vi "ScientiFic DC Power Supply Output DC Volts.vi"() -> ()   [LabVIEW 2020]
doc: "This example shows how to configure the instrument's output voltage level, over current protection, and over voltage protection. The actual voltage level and actual current level are returned as well as whether over voltage protection (OVP) or over current protection (OCP) has been tripped."
uses:
  <instrlib>/ScientiFic DC Power Supply/Public/Ch Selector.ctl
  <instrlib>/ScientiFic DC Power Supply/ScientiFic DC Power Supply.lvlib
panel:
  in  "Ch Selector":T1
  in  "Serial Configuration":T2={"Baud Rate"=9600, "Parity"=0, "Data Bits"=8, "Stop Bits"=10, "Flow Control"=0, "Remote Channel"="CH 1"} {"Flow Control" items=["None", "XON/XOFF", "RTS/CTS", "XON/XOFF & RTS/CTS", "DTR/DSR", "XON/XOFF & DTR/DSR"]; "Stop Bits" items=["1.0"=10, "1.5"=15, "2.0"=20]; "Data Bits" items=["7"=7, "8"=8]; "Parity" items=["None", "Odd", "Even", "Mark", "Space"]; "Baud Rate" items=["300"=300, "600"=600, "1200"=1200, "2400"=2400, "4800"=4800, "9600"=9600, "19200"=19200]}
  in  "Stop Output":bool
  in  "Voltage Set (0V)":dbl format="%.2f"
  out "Actual Current Limit (A)":dbl format="%.2f"
  out "Actual Voltage Level (V)":dbl format="%.2f"
  in  "Current Set (0A)":dbl format="%.2f"
  in  "VISA resource name":refnum<visa-resource-name>
  # "(c) 2021 <ScientiFic Mes Technik Pvt Ltd>.  ALL RIGHTS RESERVED."
  # "Serial Configuration"
  # "Set Voltage"
  # "Set Current"
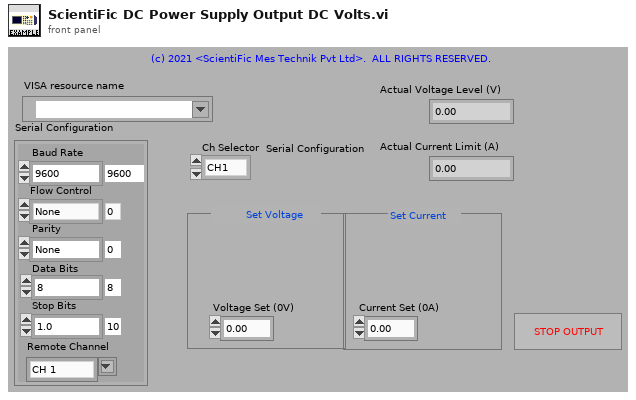
[diagram p1: front panel]
types:
  T1 = typedef "ScientiFic DC Power Supply.lvlib/Ch Selector.ctl" = enum16{"CH1", "CH2", "CH3", "CH4"}
  T2 = cluster{"Baud Rate":u32, "Parity":u16, "Data Bits":u16, "Stop Bits":u16, "Flow Control":u16, "Remote Channel":string}
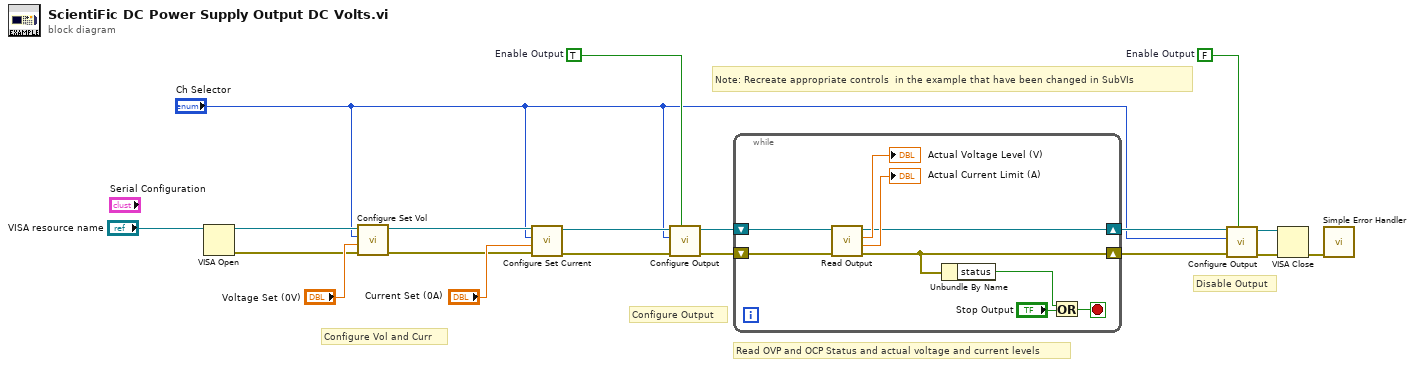
[diagram p0: block diagram]
diagram:
  w10 = FALSE  # Enable Output
  w11 = TRUE  # Enable Output
  # "Note: Recreate appropriate controls  in the example that have been changed in SubVIs"
  # "Disable Output"
  # "Read OVP and OCP Status and actual voltage and current levels"
  # "Configure Output"
  # "Configure Vol and Curr"
  n1 = VISA Open(VISA resource name="VISA resource name") -> (VISA resource name=w4:refnum<visa-resource-name>, error out=w3:errorcluster)  [unwired: 4 in]
  n2 = call <instrlib>:"Configure Set Vol.vi"("error in (no error)"=w3, "Voltage set (0.00 V)"="Voltage Set (0V)", "Ch Selector"="Ch Selector", "VISA resource name"=w4) -> ("error out"=w5:errorcluster, "VISA resource name out"=w6:refnum<visa-resource-name>)  [unwired: 6 in]
  n3 = call <instrlib>:"Configure Set Current.vi"("error in (no error)"=w5, "Current Set (0.0 A)"="Current Set (0A)", "Ch Selector"="Ch Selector", "VISA resource name"=w6) -> ("error out"=w18:errorcluster, "VISA resource name out"=w19:refnum<visa-resource-name>)  [unwired: 6 in]
  n4 = call <instrlib>:"Configure Output.vi"("Enable Output (T: Enable)"=w11, "error in (no error)"=w18, "Ch Selector"="Ch Selector", "VISA resource name"=w19) -> ("error out"=w16:errorcluster, "VISA resource name out"=w17:refnum<visa-resource-name>)  [unwired: 6 in]
  n5 = while {
    shift-right: [w24] -> w15
    shift-left: w16 -> [w21]
    shift-right: [w20] -> w7
    shift-left: w17 -> [w22]
    stop <- w26 stop-if-true
    n6 = call <instrlib>:"Read Output.vi"("error in (no error)"=w21, "VISA resource name"=w22) -> ("error out"=w24:errorcluster, "Actual Current Level (A)"=→"Actual Current Limit (A)":dbl, "Actual Voltage Level (V)"=→"Actual Voltage Level (V)":dbl, "VISA resource name out"=w20:refnum<visa-resource-name>)  [unwired: 6 in]
    n7 = Unbundle By Name(w24) -> ("status"=w23:bool)
    n8 = Or(x=w23, y="Stop Output") -> (x .or. y?=w26:bool)
  }
  n9 = call <instrlib>:"Configure Output.vi"("Enable Output (T: Enable)"=w10, "error in (no error)"=w15, "Ch Selector"="Ch Selector", "VISA resource name"=w7) -> ("error out"=w13:errorcluster, "VISA resource name out"=w14:refnum<visa-resource-name>)  [unwired: 6 in]
  n10 = VISA Close(VISA resource name=w14, error in (no error)=w13) -> (error out=w9:errorcluster)
  n11 = call <vilib>:"Simple Error Handler.vi"("error in (no error)"=w9) -> ()  [unwired: 4 in, 5 out]
